vi "Attempt Connect.vi"(8 "error in (no error)":errorcluster, 11 "Sift Client in":refnum<class "Sift Client.lvclass">) -> (0 "error out":errorcluster, 1 "Success":bool, 2 "Connection ID":refnum<k5>, 3 "Sift Client out":refnum<class "Sift Client.lvclass">)   [LabVIEW 2024, in "Sift Client.lvlib" / "Sift Client.lvclass"]
uses:
  Sift Client.lvclass
  Sift Client.lvclass/Sift Client.ctl
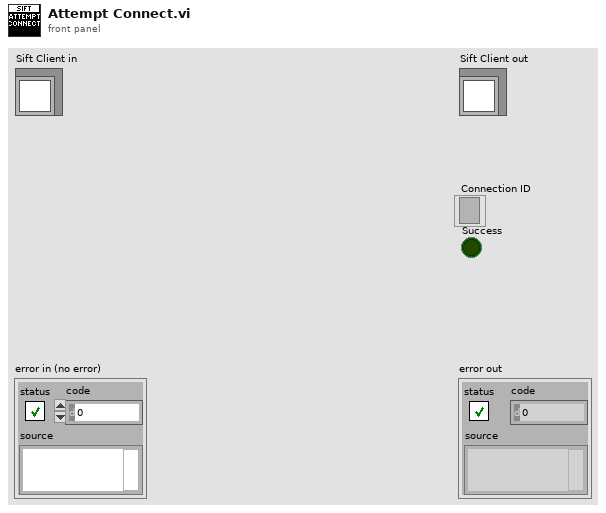
[diagram p1: front panel]
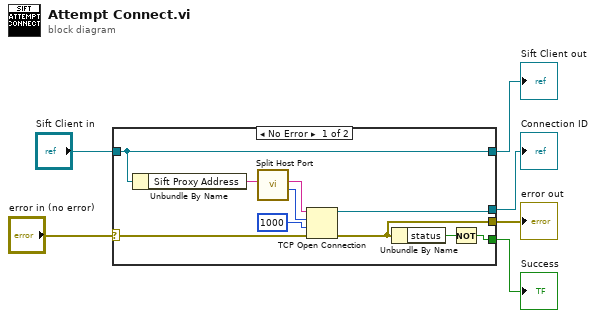
[diagram p0: block diagram]
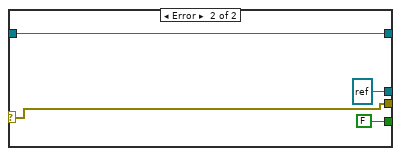
[diagram p2: hidden frame]
diagram:
  n1 = case shown="No Error" "error in (no error)" {
    selector: "error in (no error)" -> [w11 w20]
    tunnel: [w7 w20] -> w5
    tunnel: [w12 w19] -> w3
    tunnel: "Sift Client in" -> [w12 w19]
    tunnel: [w9 refnum<k5> refnum ("connection ID")] -> w2
    tunnel: [w8 FALSE] -> w1
    frame No Error {
      n2 = Unbundle By Name(w12) -> ("Sift Proxy Address"=w15:string)
      n3 = call "Split Host Port.vi"("Address"=w15) -> ("Port"=w13:i32, "Hostname"=w14:string)  [unwired: 9 in]
      n4 = TCP Open Connection(address=w14, remote port or service name=w13, timeout ms (60000)=1000, error in (no error)=w11) -> (connection ID=w9:refnum<k5>, error out=w7:errorcluster)  [unwired: 1 in]
      n5 = Unbundle By Name(w7) -> ("status"=w16:bool)
      n6 = Not(x=w16) -> (.not. x?=w8:bool)
    }
    frame Error {
    }
  }
  "error out" <- w5
  "Sift Client out" <- w3
  "Connection ID" <- w2
  "Success" <- w1
